vi "rvc Skew-Symmetric Matrix.vi"(11 "vector":dbl[](array[numeric])=[0.0, 0.0, 1.0]) -> (3 "output variable":dbl[][](array[numeric]))   [LabVIEW 2013]
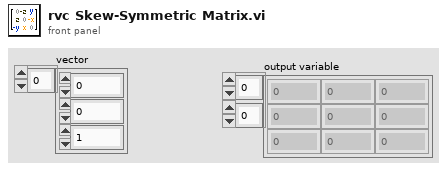
[diagram p1: front panel]
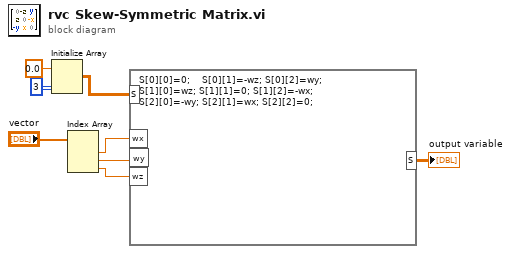
[diagram p0: block diagram]
diagram:
  w2 = 3 ("dimension size")
  n1 = Initialize Array(0.0 ("element"), w2, w2) -> (w4:dbl[][])
  n2 = Index Array(array="vector") -> (element #1=w7:dbl, element #2=w6:dbl, element #3=w5:dbl)  [unwired: 3 in]
  n3 = formula code="S[0][0]=0;    S[0][1]=-wz; S[0][2]=wy;\nS[1][0]=wz; S[1][1]=0; S[1][2]=-wx;\nS[2][0]=-wy; S[2][1]=wx; S[2][2]=0;"("wx"=w7, "wy"=w6, "wz"=w5, "S"=w4) -> ("S"=→"output variable":dbl[][])
